vi "Motors Status Verbose.vi"(5 "Axis":i32, 9 "VISA in":refnum<visa-resource-name>, 11 "error in":errorcluster) -> (1 "Slew Speed (mm or deg/s)":dbl, 2 "Jogger Normal Speed (mm or deg/s)":dbl, 3 "Jogger Fast Speed (mm or deg/s)":dbl, 4 "Actual Position (mm or deg)":dbl, 6 "OS":i32, 8 "Mode":string, 10 "VISA out":refnum<visa-resource-name>, 12 "Creep Speed (mm or deg/s)":dbl, 15 "error out":errorcluster)   [LabVIEW 2018]
panel:
  out "Creep buffer":string
  out "Slew buffer":string
  out "Actual Position buffer":string
  out "Mode buffer":string
  out "Jogger buffer":string
  out "OS buffer":string
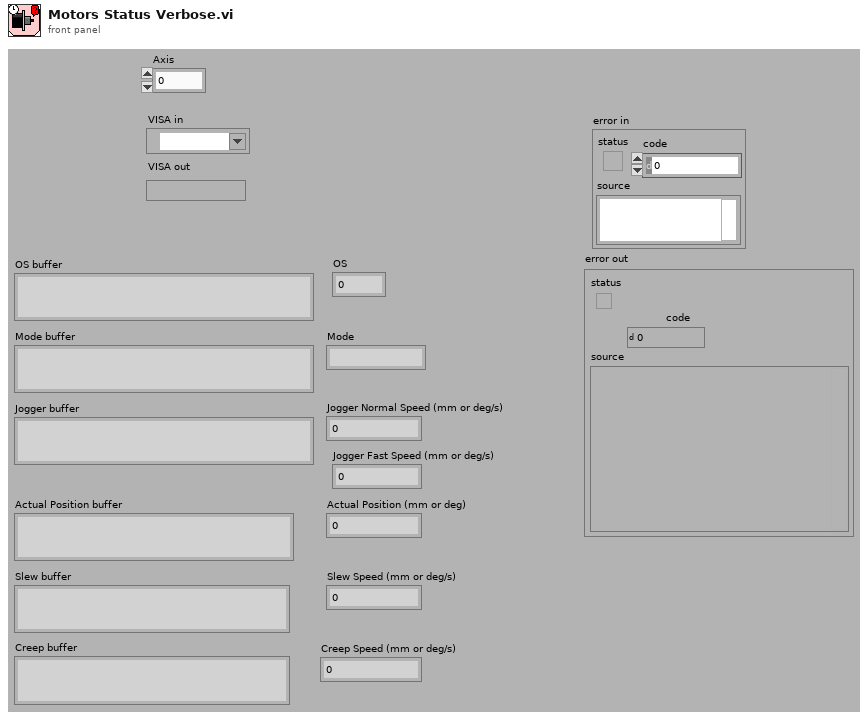
[diagram p1: front panel]
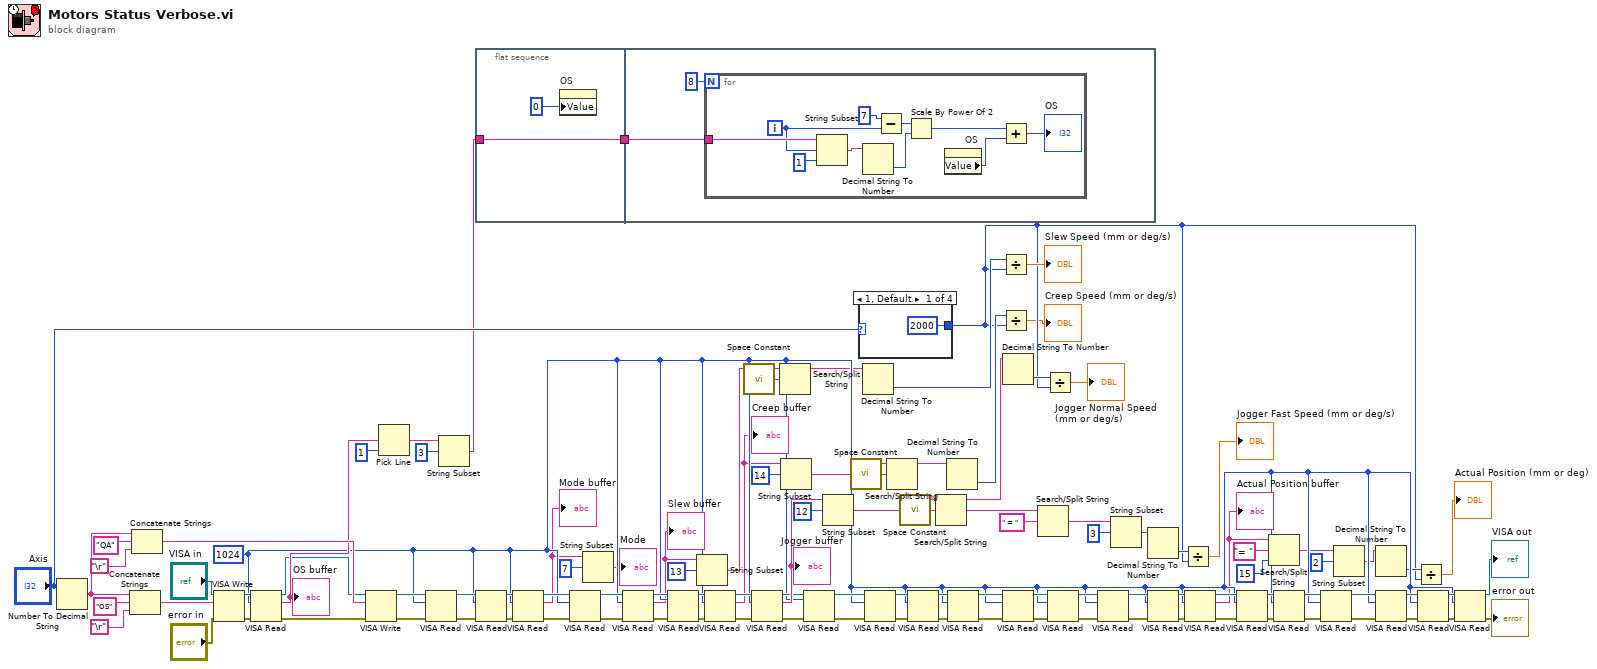
[diagram p0: block diagram]
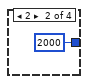
[diagram p2: hidden frame]
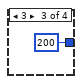
[diagram p3: hidden frame]
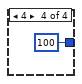
[diagram p4: hidden frame]
diagram:
  w49 = u32 1024 ("byte count")
  n1 = Number To Decimal String(number="Axis") -> (decimal integer string=w96:string)  [unwired: 1 in]
  n2 = Concatenate Strings(w96, "OS" ("Initial command 1"), "\r") -> (w103:string)
  n3 = Concatenate Strings(w96, "QA" ("Initial command 1"), "\r") -> (w102:string)
  n4 = VISA Write(VISA resource name="VISA in", write buffer=w103, error in (no error)="error in") -> (VISA resource name out=w109:refnum<visa-resource-name>, error out=w108:errorcluster)  [unwired: 1 out]
  n5 = VISA Read(VISA resource name=w109, byte count=w49, error in (no error)=w108) -> (VISA resource name out=w31:refnum<visa-resource-name>, read buffer=w100:string, error out=w32:errorcluster)  [unwired: 1 out]
  "OS buffer" <- w100
  n6 = VISA Write(VISA resource name=w31, write buffer=w102, error in (no error)=w32) -> (VISA resource name out=w106:refnum<visa-resource-name>, error out=w107:errorcluster)  [unwired: 1 out]
  n7 = Pick Line(multi-line string=w100, line index=1) -> (output string=w99:string)  [unwired: 1 in]
  n8 = VISA Read(VISA resource name=w106, byte count=w49, error in (no error)=w107) -> (VISA resource name out=w94:refnum<visa-resource-name>, error out=w93:errorcluster)  [unwired: 2 out]
  n9 = String Subset(string=w99, offset (0)=3) -> (substring=w17:string)  [unwired: 1 in]
  n10 = flat-sequence {
    tunnel: w17 -> [w111]
    tunnel: [w111] -> w16
    tunnel: w16 -> [w113]
    frame #0 {
      n11 = property on="OS" class="DigNum (strict)"("Value"=0 ("OS")) -> ()  [unwired: 2 in, 2 out]
    }
    frame #1 {
      n12 = for {
        N: 8 -> [_]
        tunnel: w113 -> [w122]
        i -> [w117]
        n13 = String Subset(string=w122, offset (0)=w117, length (rest)=1 ("length (rest)")) -> (substring=w121:string)
        n14 = Decimal String To Number(string=w121) -> (number=w120:i32)  [unwired: 2 in, 1 out]
        n15 = Subtract(x=7, y=w117) -> (x-y=w119:i32)
        n16 = Scale By Power Of 2(n=w119, x=w120) -> (x*2^n=w116:i32)
        n17 = property on="OS" class="DigNum (strict)"() -> ("Value"=w114:i32)  [unwired: 2 in, 2 out]
        n18 = Add(x=w116, y=w114) -> (x+y=→"OS":i32)
      }
    }
  }
  n19 = VISA Read(VISA resource name=w94, byte count=w49, error in (no error)=w93) -> (VISA resource name out=w90:refnum<visa-resource-name>, error out=w89:errorcluster)  [unwired: 2 out]
  n20 = VISA Read(VISA resource name=w90, byte count=w49, error in (no error)=w89) -> (VISA resource name out=w91:refnum<visa-resource-name>, read buffer=w30:string, error out=w92:errorcluster)  [unwired: 1 out]
  "Mode buffer" <- w30
  n21 = VISA Read(VISA resource name=w91, byte count=w49, error in (no error)=w92) -> (VISA resource name out=w88:refnum<visa-resource-name>, error out=w87:errorcluster)  [unwired: 2 out]
  n22 = String Subset(string=w30, offset (0)=7) -> (substring=→"Mode":string)  [unwired: 1 in]
  n23 = VISA Read(VISA resource name=w88, byte count=w49, error in (no error)=w87) -> (VISA resource name out=w86:refnum<visa-resource-name>, read buffer=w15:string, error out=w85:errorcluster)  [unwired: 1 out]
  "Slew buffer" <- w15
  n24 = VISA Read(VISA resource name=w86, byte count=w49, error in (no error)=w85) -> (VISA resource name out=w84:refnum<visa-resource-name>, error out=w82:errorcluster)  [unwired: 2 out]
  n25 = String Subset(string=w15, offset (0)=13) -> (substring=w13:string)  [unwired: 1 in]
  n26 = VISA Read(VISA resource name=w84, byte count=w49, error in (no error)=w82) -> (VISA resource name out=w83:refnum<visa-resource-name>, read buffer=w8:string, error out=w81:errorcluster)  [unwired: 1 out]
  "Creep buffer" <- w8
  n27 = call <vilib>:"Space Constant.vi"() -> ("String"=w12:string)
  n28 = VISA Read(VISA resource name=w83, byte count=w49, error in (no error)=w81) -> (VISA resource name out=w63:refnum<visa-resource-name>, read buffer=w80:string, error out=w48:errorcluster)  [unwired: 1 out]
  "Jogger buffer" <- w80
  n29 = Search/Split String(string=w13, search string/char (-)=w12) -> (substring before match=w11:string)  [unwired: 1 in, 2 out]
  n30 = String Subset(string=w8, offset (0)=14) -> (substring=w6:string)  [unwired: 1 in]
  n31 = VISA Read(VISA resource name=w63, byte count=w49, error in (no error)=w48) -> (VISA resource name out=w66:refnum<visa-resource-name>, error out=w67:errorcluster)  [unwired: 2 out]
  n32 = String Subset(string=w80, offset (0)=12) -> (substring=w78:string)  [unwired: 1 in]
  n33 = call <vilib>:"Space Constant.vi"() -> ("String"=w5:string)
  n34 = case shown="1, Default" "Axis" {
    tunnel: [2000 2000 200 100] -> w2
    frame 1, Default {
    }
    frame 2 {
    }
    frame 3 {
    }
    frame 4 {
    }
  }
  n35 = Decimal String To Number(string=w11) -> (number=w10:i32)  [unwired: 2 in, 1 out]
  n36 = VISA Read(VISA resource name=w66, byte count=w49, error in (no error)=w67) -> (VISA resource name out=w62:refnum<visa-resource-name>, error out=w47:errorcluster)  [unwired: 2 out]
  n37 = Search/Split String(string=w6, search string/char (-)=w5) -> (substring before match=w4:string)  [unwired: 1 in, 2 out]
  n38 = call <vilib>:"Space Constant.vi"() -> ("String"=w77:string)
  n39 = VISA Read(VISA resource name=w62, byte count=w49, error in (no error)=w47) -> (VISA resource name out=w61:refnum<visa-resource-name>, error out=w46:errorcluster)  [unwired: 2 out]
  n40 = Search/Split String(string=w78, search string/char (-)=w77) -> (substring before match=w72:string, match + rest of string=w73:string)  [unwired: 1 in, 1 out]
  n41 = Decimal String To Number(string=w4) -> (number=w3:i32)  [unwired: 2 in, 1 out]
  n42 = VISA Read(VISA resource name=w61, byte count=w49, error in (no error)=w46) -> (VISA resource name out=w60:refnum<visa-resource-name>, error out=w45:errorcluster)  [unwired: 2 out]
  n43 = Divide(x=w10, y=w2) -> (x/y=→"Slew Speed (mm or deg/s)":dbl)
  n44 = Divide(x=w3, y=w2) -> (x/y=→"Creep Speed (mm or deg/s)":dbl)
  n45 = Decimal String To Number(string=w72) -> (number=w70:i32)  [unwired: 2 in, 1 out]
  n46 = VISA Read(VISA resource name=w60, byte count=w49, error in (no error)=w45) -> (VISA resource name out=w59:refnum<visa-resource-name>, error out=w44:errorcluster)  [unwired: 2 out]
  n47 = Search/Split String(string=w73, search string/char (-)=" = ") -> (match + rest of string=w75:string)  [unwired: 1 in, 2 out]
  n48 = Divide(x=w70, y=w2) -> (x/y=→"Jogger Normal Speed (mm or deg/s)":dbl)
  n49 = VISA Read(VISA resource name=w59, byte count=w49, error in (no error)=w44) -> (VISA resource name out=w58:refnum<visa-resource-name>, error out=w43:errorcluster)  [unwired: 2 out]
  n50 = VISA Read(VISA resource name=w58, byte count=w49, error in (no error)=w43) -> (VISA resource name out=w57:refnum<visa-resource-name>, error out=w42:errorcluster)  [unwired: 2 out]
  n51 = String Subset(string=w75, offset (0)=3) -> (substring=w71:string)  [unwired: 1 in]
  n52 = Decimal String To Number(string=w71) -> (number=w69:i32)  [unwired: 2 in, 1 out]
  n53 = VISA Read(VISA resource name=w57, byte count=w49, error in (no error)=w42) -> (VISA resource name out=w56:refnum<visa-resource-name>, error out=w41:errorcluster)  [unwired: 2 out]
  n54 = Divide(x=w69, y=w2) -> (x/y=→"Jogger Fast Speed (mm or deg/s)":dbl)
  n55 = VISA Read(VISA resource name=w56, byte count=w49, error in (no error)=w41) -> (VISA resource name out=w55:refnum<visa-resource-name>, read buffer=w27:string, error out=w40:errorcluster)  [unwired: 1 out]
  "Actual Position buffer" <- w27
  n56 = VISA Read(VISA resource name=w55, byte count=w49, error in (no error)=w40) -> (VISA resource name out=w54:refnum<visa-resource-name>, error out=w39:errorcluster)  [unwired: 2 out]
  n57 = Search/Split String(string=w27, search string/char (-)="= ", offset (0)=15) -> (match + rest of string=w24:string)  [unwired: 2 out]
  n58 = VISA Read(VISA resource name=w54, byte count=w49, error in (no error)=w39) -> (VISA resource name out=w64:refnum<visa-resource-name>, error out=w65:errorcluster)  [unwired: 2 out]
  n59 = VISA Read(VISA resource name=w64, byte count=w49, error in (no error)=w65) -> (VISA resource name out=w53:refnum<visa-resource-name>, error out=w38:errorcluster)  [unwired: 2 out]
  n60 = String Subset(string=w24, offset (0)=2) -> (substring=w22:string)  [unwired: 1 in]
  n61 = Decimal String To Number(string=w22) -> (number=w21:i32)  [unwired: 2 in, 1 out]
  n62 = VISA Read(VISA resource name=w53, byte count=w49, error in (no error)=w38) -> (VISA resource name out=w52:refnum<visa-resource-name>, error out=w37:errorcluster)  [unwired: 2 out]
  n63 = Divide(x=w21, y=w2) -> (x/y=→"Actual Position (mm or deg)":dbl)
  n64 = VISA Read(VISA resource name=w52, byte count=w49, error in (no error)=w37) -> (VISA resource name out=w51:refnum<visa-resource-name>, error out=w36:errorcluster)  [unwired: 2 out]
  n65 = VISA Read(VISA resource name=w51, byte count=w49, error in (no error)=w36) -> (VISA resource name out=→"VISA out":refnum<visa-resource-name>, error out=→"error out":errorcluster)  [unwired: 2 out]
